vi "tcp read.vi"(7 "Connection in":refnum<k5>, 8 "error in":errorcluster) -> (0 "error out":errorcluster, 2 "Data":string)   [LabVIEW 2013]
doc: "# #############################################################################\n# ATTENTION\n# #############################################################################\n#\n# This software is for guidance only. It is provided \"as is\".\n# It only aims at providing coding information to the customer in order for\n# them to save time. As a result no warranties, whether express, implied or\n# statutory, including, but not limited to implied warranties of\n# merchantability and fitness for a particular purpose apply to this software.\n# A·P·E Angewandte Physik und Elektronik GmbH shall not be held liable for any\n# direct, indirect or consequential damages with respect to any claims arising\n# from the content of such sourcecode and/or the use made by customers of the\n# coding information contained herein in connection with their products.\n#\n# #############################################################################"
uses:
  <vilib>/regexp/Match Regular Expression.xnode
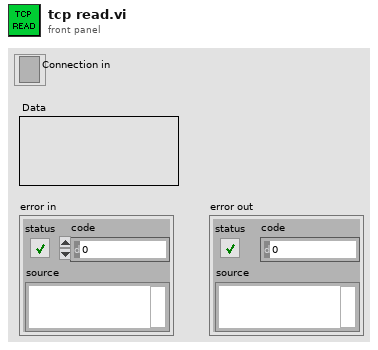
[diagram p1: front panel]
types:
  T1 = enum16{"Standard", "Buffered", "CRLF", "Immediate"}
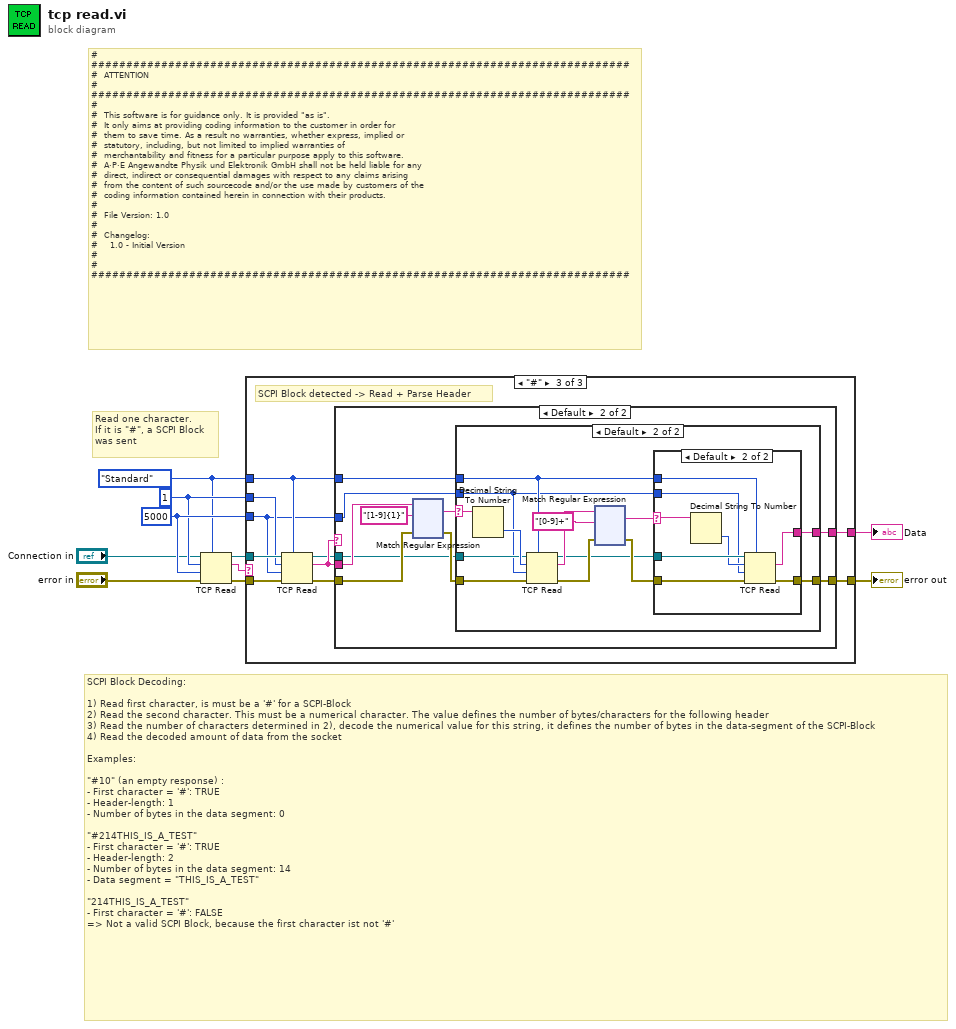
[diagram p0: block diagram]
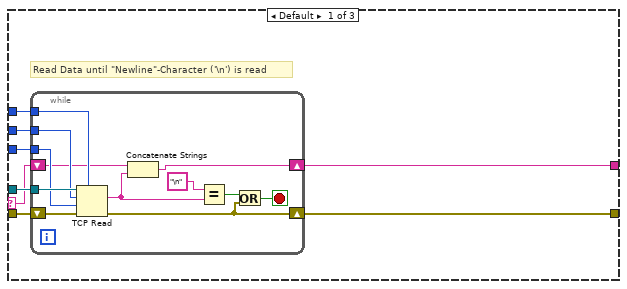
[diagram p2: hidden frame]
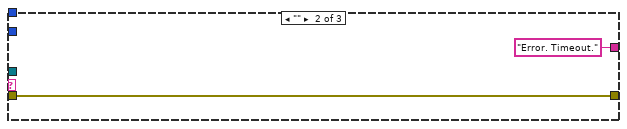
[diagram p3: hidden frame]
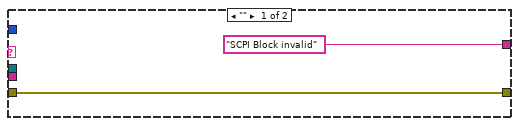
[diagram p4: hidden frame]
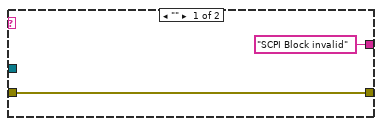
[diagram p5: hidden frame]
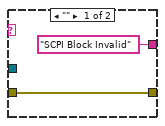
[diagram p6: hidden frame]
diagram:
  w10 = 5000 ("timeout ms (25000)")
  w9 = 1 ("bytes to read")
  w8 = T1."Standard" ("mode (standard)")
  # "# #############################################################################\n#  ATTENTION\n# #############################################################################\n#\n#  This software is for guidance only. It is provided \"as is\".\n#  It only aims at providing coding information to the customer in order for\n#  them to save time. As a result no warranties, whether express, implied or\n#  statutory, including, but not limited to implied warranties of\n#  merchantability and fitness for a particular purpose apply to this software.\n#  A·P·E Angewandte Physik und Elektronik GmbH shall not be held liable for any\n#  direct, indirect or consequential damages with respect to any claims arising\n#  from the content of such sourcecode and/or the use made by customers of the\n#  coding information contained herein in connection with their products.\n#\n#  File Version: 1.0\n#\n#  Changelog:\n#    1.0 - Initial Version\n#\n# #############################################################################"
  # "SCPI Block Decoding:\n\n1) Read first character, is must be a '#' for a SCPI-Block\n2) Read the second character. This must be a numerical character. The value defines the number of bytes/characters for the following header\n3) Read the number of characters determined in 2), decode the numerical value for this string, it defines the number of bytes in the data-segment of the SCPI-Block\n4) Read the decoded amount of data from the socket\n\nExamples:\n\n\"#10\" (an empty response) :\n- First character = '#': TRUE\n- Header-length: 1\n- Number of bytes in the data segment: 0\n\n\"#214THIS_IS_A_TEST\" \n- First character = '#': TRUE\n- Header-length: 2\n- Number of bytes in the data segment: 14\n- Data segment = \"THIS_IS_A_TEST\"\n\n\"214THIS_IS_A_TEST\"\n- First character = '#': FALSE\n=> Not a valid SCPI Block, because the first character ist not '#'"
  # "Read one character.\nIf it is \"#\", a SCPI Block \nwas sent"
  n1 = TCP Read(connection ID="Connection in", bytes to read=w9, error in (no error)="error in", 7:w8, 9:w10) -> (connection ID out=w7:refnum<k5>, data out=w6:string, error out=w5:errorcluster)
  n2 = case shown="\"#\"" w6 {
    selector: w6 -> [w12 _ _]
    tunnel: w5 -> [w18 w31 w42]
    tunnel: [w17 w31 w37] -> w4
    tunnel: w7 -> [w16 _ w41]
    tunnel: w8 -> [w15 _ w34]
    tunnel: w9 -> [w14 _ w40]
    tunnel: w10 -> [w13 _ w33]
    tunnel: [w11 "Error. Timeout." ("data out") w36] -> w1
    frame Default {
      # "Read Data until \"Newline\"-Character ('\\n') is read"
      n3 = while {
        tunnel: w16 -> [w29]
        shift-right: [w19] -> w17
        shift-left: w18 -> [w30]
        tunnel: w15 -> [w28]
        tunnel: w14 -> [w27]
        tunnel: w13 -> [w26]
        shift-right: [w24] -> w11
        shift-left: w12 -> [w25]
        stop <- w20 stop-if-true
        n4 = TCP Read(connection ID=w29, bytes to read=w27, error in (no error)=w30, 7:w28, 9:w26) -> (data out=w23:string, error out=w19:errorcluster)  [unwired: 1 out]
        n5 = Concatenate Strings(w25, w23) -> (w24:string)
        n6 = Equal?(x="\n" ("y"), y=w23) -> (x = y?=w21:bool)
        n7 = Or(x=w21, y=w19) -> (x .or. y?=w20:bool)
      }
    }
    frame "" {
    }
    frame "#" {
      # "SCPI Block detected -> Read + Parse Header"
      n8 = TCP Read(connection ID=w41, bytes to read=w40, error in (no error)=w42, 7:w34, 9:w33) -> (connection ID out=w35:refnum<k5>, data out=w38:string, error out=w39:errorcluster)
      n9 = case shown="Default" w38 {
        tunnel: w39 -> [w43 w54]
        tunnel: w38 -> [_ w53]
        tunnel: [w43 w46] -> w37
        tunnel: ["SCPI Block invalid" w45] -> w36
        tunnel: w35 -> [_ w50]
        tunnel: w34 -> [_ w49]
        tunnel: w33 -> [_ w48]
        frame "" {
        }
        frame Default {
          n10 = xnode "Match Regular Expression"("input string"=w53, "regular expression"="[1-9]{1}", "error in"=w54) -> ("whole match"=w47:string, "error out"=w51:errorcluster)  [unwired: 3 in, 3 out]
          n11 = case shown="Default" w47 {
            selector: w47 -> [_ w67]
            tunnel: w51 -> [w56 w69]
            tunnel: w50 -> [_ w68]
            tunnel: w49 -> [_ w59]
            tunnel: w48 -> [_ w58]
            tunnel: [w56 w62] -> w46
            tunnel: ["SCPI Block invalid" ("data out") w57] -> w45
            frame "" {
            }
            frame Default {
              n12 = Decimal String To Number(string=w67) -> (number=w70:i32)  [unwired: 2 in, 1 out]
              n13 = TCP Read(connection ID=w68, bytes to read=w70, error in (no error)=w69, 7:w59, 9:w58) -> (connection ID out=w60:refnum<k5>, data out=w64:string, error out=w65:errorcluster)
              n14 = xnode "Match Regular Expression"("input string"=w64, "regular expression"="[0-9]+", "error in"=w65) -> ("whole match"=w61:string, "error out"=w63:errorcluster)  [unwired: 3 in, 3 out]
              n15 = case shown="Default" w61 {
                selector: w61 -> [_ w77]
                tunnel: w63 -> [w71 w80]
                tunnel: [w71 w79] -> w62
                tunnel: w60 -> [_ w78]
                tunnel: w59 -> [_ w76]
                tunnel: w58 -> [_ w74]
                tunnel: ["SCPI Block Invalid" ("data out") w73] -> w57
                frame "" {
                }
                frame Default {
                  n16 = Decimal String To Number(string=w77) -> (number=w75:i32)  [unwired: 2 in, 1 out]
                  n17 = TCP Read(connection ID=w78, bytes to read=w75, error in (no error)=w80, 7:w76, 9:w74) -> (data out=w73:string, error out=w79:errorcluster)  [unwired: 1 out]
                }
              }
            }
          }
        }
      }
    }
  }
  "error out" <- w4
  "Data" <- w1
